vi "UI Actor Launcher.vi"   [LabVIEW 2020, in "UI Actor.lvlib"]
uses:
  UI Actor.lvlib
  UI Actor/UI Actor.lvclass
  C:/Program Files (x86)/National Instruments/LabVIEW 2020/vi.lib/ActorFramework/Actor/Actor.lvclass
  <vilib>/ActorFramework/Actor/Actor.lvclass
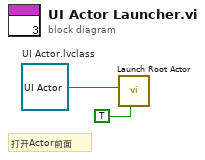
[diagram p0: block diagram]
diagram:
  w2 = refnum<class "UI Actor.lvclass"> refnum  # UI Actor.lvclass
  # "打开Actor前面"
  n1 = call <vilib>:"Launch Root Actor.vi"("Open Actor Core front panel? (F)"=TRUE, "Actor"=w2) -> ()  [unwired: 8 in, 2 out]
